vi "Demo_CreateMovie.vi"() -> ()   [LabVIEW 2024]
doc: "Create a video movie made of LV images. The images can be compressed.\n\n© Chris Salzmann, 1994-2003"
uses:
  <userlib>/ImageProcessing/QTLIB_2595_LV86/QT_Private.ctl
  <userlib>/ImageProcessing/QTLIB_2595_LV86/QT_File.ctl
  <userlib>/ImageProcessing/QTLIB_2595_LV86/QT_Compression.ctl
  <userlib>/ImageProcessing/QTLIB_2595_LV86/QT_Movie.ctl
panel:
  in  "Frame duration [ms]":i32
  in  "Compression":i32(slide) scale=0.0..1024.0 scale format="%.0x"
  in  "Format":u16(ring) items=["Animation ' elr'", "Apple Intermediate Codec 'doci'", "Apple Pixlet Video 'tlxp'", "BMP 'ELRW'", "Cinepak 'divc'", "Component Video '2vuy'", "DV - PAL 'pcvd'", "DV/DVCPRO - NTSC ' cvd'", "DVCPRO - PAL 'ppvd'", "DVCPRO50 - NTSC 'n5vd'", "DVCPRO50 - PAL 'p5vd'", "Graphics ' cms'", "H.261 '162h'", "H.263 '362h'", "H.264 '1cva'", "JPEG 2000 '2pjm'", "Motion JPEG A 'apjm'", "Motion JPEG B 'bpjm'", "MPEG-4 Video 'v4pm'", "None ' war'", "Photo - JPEG 'gepj'", "Planar RGB 'SPB8'", "PNG ' gnp'", "Sorenson Video '1QVS'", "Sorenson Video 3 '3QVS'", "TGA ' agt'", "TIFF 'ffit'", "Video 'azpr'"]
  out "Current Frame":picture
  out "error out":errorcluster={"status"=TRUE, "code"=-43, "source"=""}
  in  "stop":bool
  in  "Movie Settings":T1={"Width"=100, "Height"=100, "Time Base"=1000, "Type"=0, "Creator"=0, "Flatten"=0, "Options"=0, "Author"="Chris", "Information"="from LV Qt tlbx", "Copyright"="©94-2002", "Dialogs"=0} {"Dialogs" format="%.0b"}
  in  "Max Nbr Frames in the movie":i32=1
  in  "Movie path":path=path "Y:/pc2.mov"
  # "Create a video movie made of LV images. The images can be compressed.\n\n© Chris Salzmann, 1994-2005"
  # "Amination is lossless\nJPEG provides hight compression\nNo temporal compression at this time!"
  # "Min"
  # "Normal"
  # "Loss less"
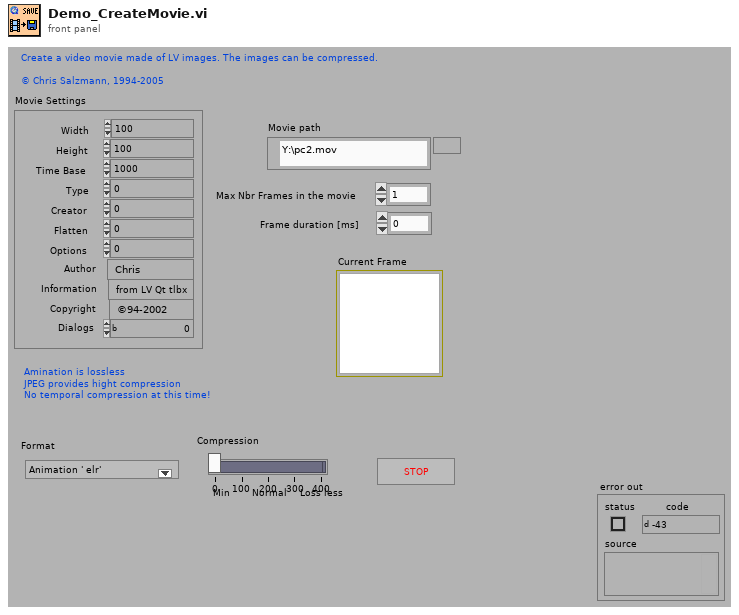
[diagram p1: front panel]
types:
  T1 = typedef "QT_Movie.ctl" = cluster{"Width":i32, "Height":i32, "Time Base":i32, "Type":i32, "Creator":i32, "Flatten":i32, "Options":i32, "Author":string, "Information":string, "Copyright":string, "Dialogs":u32}
  T2 = typedef "QT_Compression.ctl" = cluster{"Compression":i32, "Format":i32, "Codec":i32, "Comp. Quality":i32, "Key Frame":i32, "Dialogs":u32}
  T3 = typedef "QT_File.ctl" = cluster{"Paths":string[], "Options":i32, "Dialogs":u32, "Reserved":i32}
  T4 = typedef "QT_Private.ctl" = cluster{"reserved 1":i32, "reserved 2":i32, "reserved 3":i32, "reserved 4":i32}
  T5 = typedef "QT_Ref.ctl" = refnum<k1>
  T6 = typedef "QT_Image.ctl" = cluster{"Width":i32, "Height":i32, "Depth":i32, "data":u8[], "Compressed data":u8[], "Color table":u32[], "Duration":i32, "Options":i32, "Timestamp":i32, "ID":i32, "Reserved":i32, "Dialogs":u32}
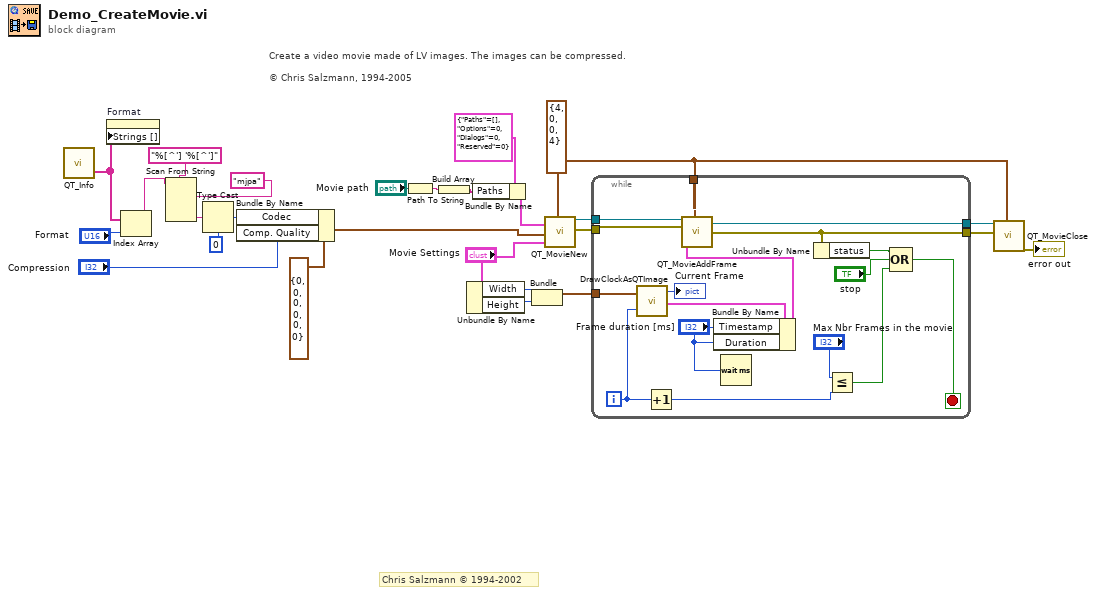
[diagram p0: block diagram]
diagram:
  w19 = T4 {"reserved 1"=4, "reserved 2"=0, "reserved 3"=0, "reserved 4"=4} ("Private")
  # "Create a video movie made of LV images. The images can be compressed.\n\n© Chris Salzmann, 1994-2005"
  # "Chris Salzmann © 1994-2002"
  n1 = call <userlib>:"QT_Info.vi"() -> ("Codec"=w5:string[])  [unwired: 3 in, 16 out]
  n2 = property on="Format" class="Ring (strict)"("Strings []"=w5) -> ()  [unwired: 2 in, 2 out]
  n3 = Index Array(array=w5, index="Format") -> (element=w4:string)
  n4 = Scan From String(format string="%[^'] '%[^']", input string=w4) -> ()  [unwired: 2 in, 7 out]
  n5 = Type Cast(type=0 ("Format"), x="mjpa" ("format string")) -> (*(type *) &x=w11:i32)
  n6 = Bundle By Name(cluster=T2 {"Compression"=0, "Format"=0, "Codec"=0, "Comp. Quality"=0, "Key Frame"=0, "Dialogs"=0} ("Compression Settings"), "Codec"=w11, "Comp. Quality"="Compression") -> (w6:T2)
  n7 = Path To String(path="Movie path") -> (string=w24:string)
  n8 = Build Array(w24) -> (w2:string[])
  n9 = Unbundle By Name("Movie Settings") -> ("Width"=w14:i32, "Height"=w13:i32)
  n10 = Bundle By Name(cluster=T3 {"Paths"=[], "Options"=0, "Dialogs"=0, "Reserved"=0} ("File Settings"), "Paths"=w2) -> (w20:T3)
  n11 = Bundle("Width"=w14, "Height"=w13) -> (w12:cluster{"Width":i32, "Height":i32})  [unwired: 1 out]
  n12 = call <userlib>:"QT_MovieNew.vi"("File Settings"=w20, "Movie Settings"="Movie Settings", "Compression Settings"=w6, "Private"=w19) -> ("QT Ref Out"=w22:T5, "error out"=w18:errorcluster)  [unwired: 2 in, 12 out]
  n13 = while {
    tunnel: w12 -> [w27]
    tunnel: [w36] -> w17
    tunnel: w18 -> [w39]
    tunnel: w19 -> [w40]
    tunnel: [w41] -> w23
    tunnel: w22 -> [w42]
    i -> [w28]
    stop <- w32 stop-if-true
    n14 = call <userlib>:"DrawClockAsQTImage.vi"("Clock Bounds"=w27, "frame ID"=w28) -> ("Picture"=→"Current Frame":picture, "Image Out (24 bits)"=w29:T6)  [unwired: 16 out]
    n15 = Increment(x=w28) -> (x+1=w31:i32)
    n16 = Bundle By Name(cluster=w29, "Timestamp"="Frame duration [ms]", "Duration"="Frame duration [ms]") -> (w38:T6)
    n17 = call <userlib>:"QT_MovieAddFrame.vi"("QT Ref In"=w42, "Image in"=w38, "error in (no error)"=w39, "Private"=w40) -> ("QT Ref Out"=w41:T5, "error out"=w36:errorcluster)  [unwired: 1 in, 13 out]
    n18 = Wait (ms)(milliseconds to wait="Frame duration [ms]") -> ()  [unwired: 1 out]
    n19 = Unbundle By Name(w36) -> ("status"=w35:bool)
    n20 = Less Or Equal?(x="Max Nbr Frames in the movie", y=w31) -> (x <= y?=w33:bool)
    n21 = Compound Arithmetic op=OR(w35, "stop", w33) -> (w32:bool)
  }
  n22 = call <userlib>:"QT_MovieClose.vi"("QT Ref In"=w23, "error in (no error)"=w17, "Private"=w19) -> ("error out"=→"error out":errorcluster)  [unwired: 16 out]
